vi "DevScan.vi"(4 "Ïµ½y î‘B":refnum<vi>, 6 "VerifyTimes":i32, 8 "错误输入（无错误）":errorcluster, 9 "需要掃描的":refnum<vi>, 10 "ESDShower":refnum<vi>, 11 "DevControl输入":refnum<class "DevControl.lvclass">) -> (0 "error out":errorcluster caption="错误输出", 2 "有變化的部分":string)   [LabVIEW 2012]
uses:
  Fun/Dev/DevControl.lvclass
  SystemState.ctl
  Dev_State_Color.ctl
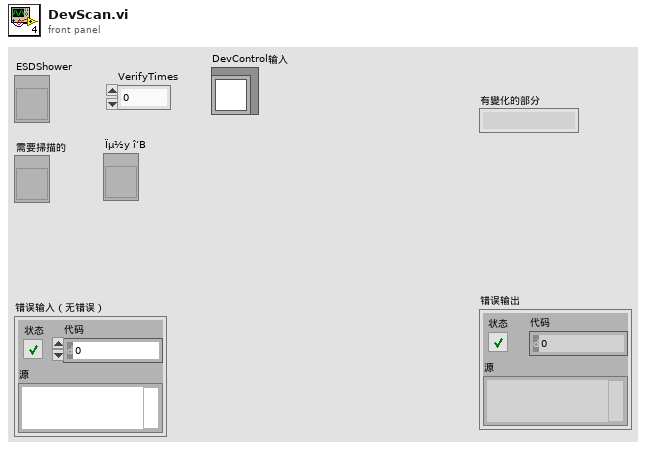
[diagram p1: front panel]
types:
  T1 = typedef "DevControl.lvclass/DevState.ctl" = enum16{"Shutdown", "PASS", "FAIL", "Idle", "Noresponse"}
  T2 = cluster{"Addr":u8, "name":string, "State":T1, "Retry":i32}[]
  T3 = typedef "SystemState.ctl" = enum16{"Quit", "Error", "Stopping", "Starting", "Init", "Scan", "Menu", "ReadConf", "Idle"}
  T4 = cluster{"Addr":u8, "name":string, "State":T1, "Retry":i32}
  T5 = typedef "Dev_State_Color.ctl" = u32
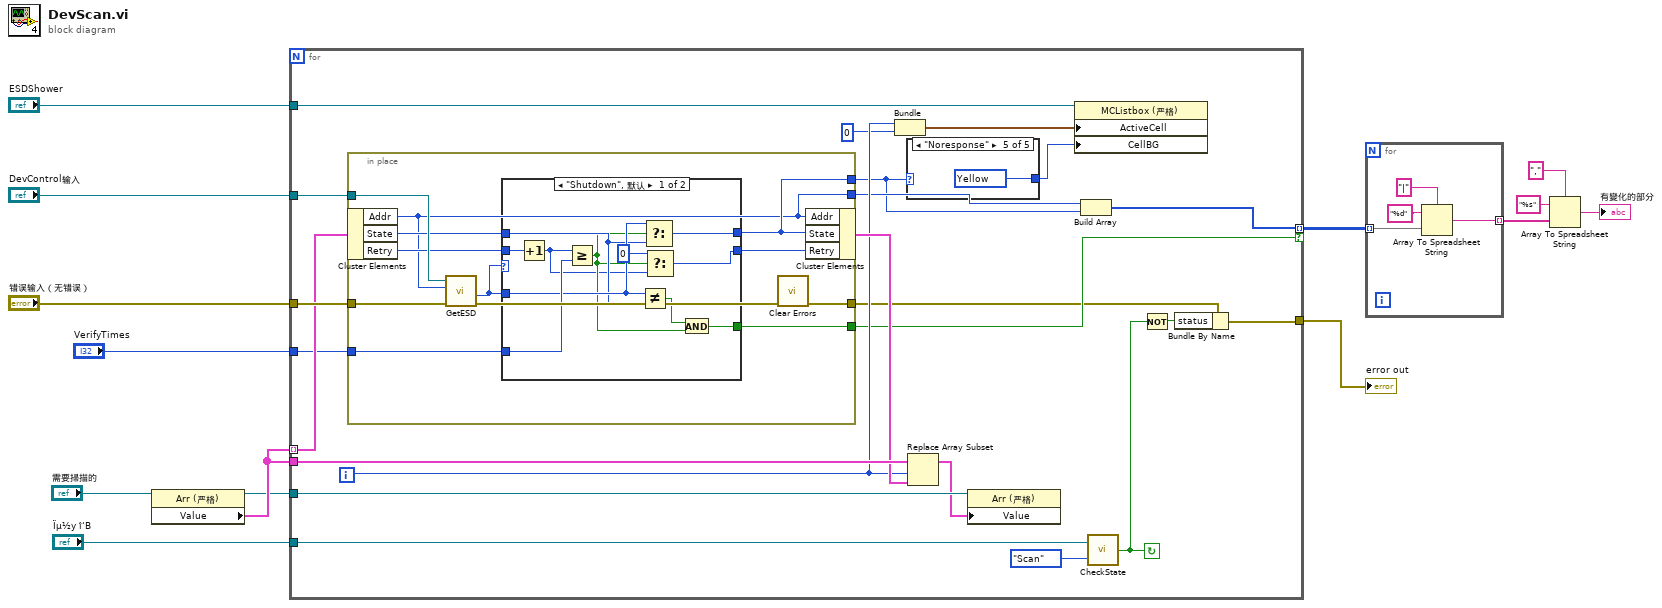
[diagram p0: block diagram]
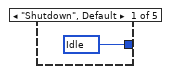
[diagram p2: hidden frame]
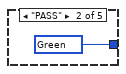
[diagram p3: hidden frame]
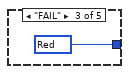
[diagram p4: hidden frame]
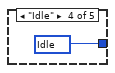
[diagram p5: hidden frame]
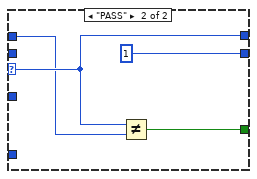
[diagram p6: hidden frame]
diagram:
  n1 = property class="Arr (严格)"(reference="需要掃描的") -> (reference out=w6:refnum<vi>, "Value"=w7:T2)  [unwired: 1 in, 1 out]
  n2 = for {
    tunnel: "DevControl输入" -> [w36]
    tunnel: "错误输入（无错误）" -> [w37]
    tunnel: w7 -> [w35] mode=indexing
    tunnel: "VerifyTimes" -> [w34]
    tunnel: "ESDShower" -> [w27]
    tunnel: "Ïµ½y î‘B" -> [w29]
    tunnel: [w18] -> w8
    tunnel: w7 -> [w33]
    tunnel: w6 -> [w31]
    tunnel: [w15] -> w5 mode=indexing if=w22
    i -> [w25]
    stop <- w19 continue-if-true
    n3 = in-place {
      in-place-border: w37 -> [w54]
      in-place-border: w36 -> [w53]
      in-place-border: w34 -> [w47]
      in-place-border: [w51] -> w21
      in-place-border: [w45] -> w16
      in-place-border: [w44] -> w17
      in-place-border: [w43] -> w22
      n4 = in-place-cluster #1(w35) -> ("Addr"=w44:u8, "State"=w48:T1, "Retry"=w50:i32)
      n5 = call-dynamic "GetESD.vi"("error in (no error)"=w54, "Addr"=w44, "DevControl 输入"=w53) -> ("error out"=w52:errorcluster, "ÑbÖÃ î‘B"=w46:T1)  [unwired: 6 in, 1 out]
      n6 = case shown="\"Shutdown\", 默认" w46 {
        selector: w46 -> [_ w68]
        tunnel: w50 -> [w65 _]
        tunnel: [w63 w68] -> w45
        tunnel: [w58 1] -> w49
        tunnel: w48 -> [w61 w67]
        tunnel: w47 -> [w64 _]
        tunnel: w46 -> [w62 _]
        tunnel: [w60 w66] -> w43
        frame "Shutdown", Default {
          n7 = Increment(x=w65) -> (x+1=w55:i32)
          n8 = Greater Or Equal?(x=w55, y=w64) -> (x >= y?=w57:bool)
          n9 = Not Equal?(x=w62, y=w61) -> (x != y?=w59:bool)
          n10 = Select(t=w62, s=w57, f=w61) -> (s? t:f=w63:T1)
          n11 = Select(t=0, s=w57, f=w55) -> (s? t:f=w58:i32)
          n12 = And(x=w59, y=w57) -> (x .and. y?=w60:bool)
        }
        frame "PASS" {
          n13 = Not Equal?(x=w68, y=w67) -> (x != y?=w66:bool)
        }
      }
      n14 = call <vilib>:"Clear Errors.vi"("error in (no error)"=w52) -> ("error out"=w51:errorcluster)  [unwired: 6 in]
      n15 = in-place-cluster #1("Addr"=w44, "State"=w45, "Retry"=w49) -> (w32:T4)
    }
    n16 = Bundle(w25, 0) -> (w26:cluster{i32, i32})  [unwired: 1 in]
    n17 = case shown="\"Noresponse\"" w16 {
      tunnel: [w38 w39 w40 w41 w42] -> w23
      frame "Shutdown", Default {
        w38 = T5 11121611 items=["Idle"=11121611, "Yellow"=16772209, "Red"=16711680, "Green"=6618880] ("DevState_Color")
      }
      frame "PASS" {
        w39 = T5 6618880 items=["Yellow"=16772209, "Red"=16711680, "Green"=6618880] ("DevState_Color")
      }
      frame "FAIL" {
        w40 = T5 16711680 items=["Yellow"=16772209, "Red"=16711680, "Green"=6618880] ("DevState_Color")
      }
      frame "Idle" {
        w41 = T5 11121611 items=["Idle"=11121611, "Yellow"=16772209, "Red"=16711680, "Green"=6618880] ("DevState_Color")
      }
      frame "Noresponse" {
        w42 = T5 16772209 items=["Yellow"=16772209, "Red"=16711680, "Green"=6618880] ("DevState_Color")
      }
    }
    n18 = Replace Array Subset(array=w33, new element=w32, index=w25) -> (w30:T2)
    n19 = property class="Arr (严格)"(reference=w31, "Value"=w30) -> ()  [unwired: 1 in, 2 out]
    n20 = property class="MCListbox (严格)"(reference=w27, "ActiveCell"=w26, "CellBG"=w23) -> ()  [unwired: 1 in, 2 out]
    n21 = Build Array(w17, w16) -> (w15:u16[])
    n22 = call "CheckState.vi"("™z²é î‘B"=SystemState."Scan", "Ïµ½y î‘B"=w29) -> ("ChkOK?"=w19:bool)
    n23 = Not(x=w19) -> (.not. x?=w20:bool)
    n24 = Bundle By Name(cluster=w21, "status"=w20) -> (w18:errorcluster)
  }
  "error out" <- w8
  n25 = for {
    tunnel: w5 -> [w73] mode=indexing
    tunnel: [w70] -> w4 mode=indexing
    n26 = Array To Spreadsheet String(delimiter (Tab)="|" ("分隔符(Tab)"), array=w73, 3:"%d" ("格式字符串")) -> (spreadsheet string=w70:string)
  }
  n27 = Array To Spreadsheet String(delimiter (Tab)="," ("分隔符(Tab)"), array=w4, 3:"%s" ("格式字符串")) -> (spreadsheet string=→"有變化的部分":string)
